vi "WILT Step Cooling Down.vi"(6 "Cool Down Period (seconds)":dbl=12.0 format="%#_13g", 7 "Station Number in":u32, 8 "Error In":errorcluster, 10 "Step 3 Input":T1, 11 "Dryer Step 5 In":T3 {"Night Cycle Count" format="%04d"; "Day Cycle Count" format="%04d"}) -> (0 "Error Out":errorcluster, 2 "Step 5 Output":T1, 3 "Dryer Step 5 Output":T3 {"Night Cycle Count" format="%04d"; "Day Cycle Count" format="%04d"})   [LabVIEW 2016]
uses:
  Type Definitions/WILT Station Test State Cluster.ctl
  Type Definitions/WILT Dryer Test State.ctl
  Type Definitions/WILT Dryer.ctl
  Type Definitions/WILT Dryer Details.ctl
  Type Definitions/WILT Agilent Channel Definition.ctl
  Type Definitions/WILT DAQ Data.ctl
  Globals/WILT Globals Main Program.vi
panel:
  # "Day"
  # "Night"
  # "Day"
  # "Night"
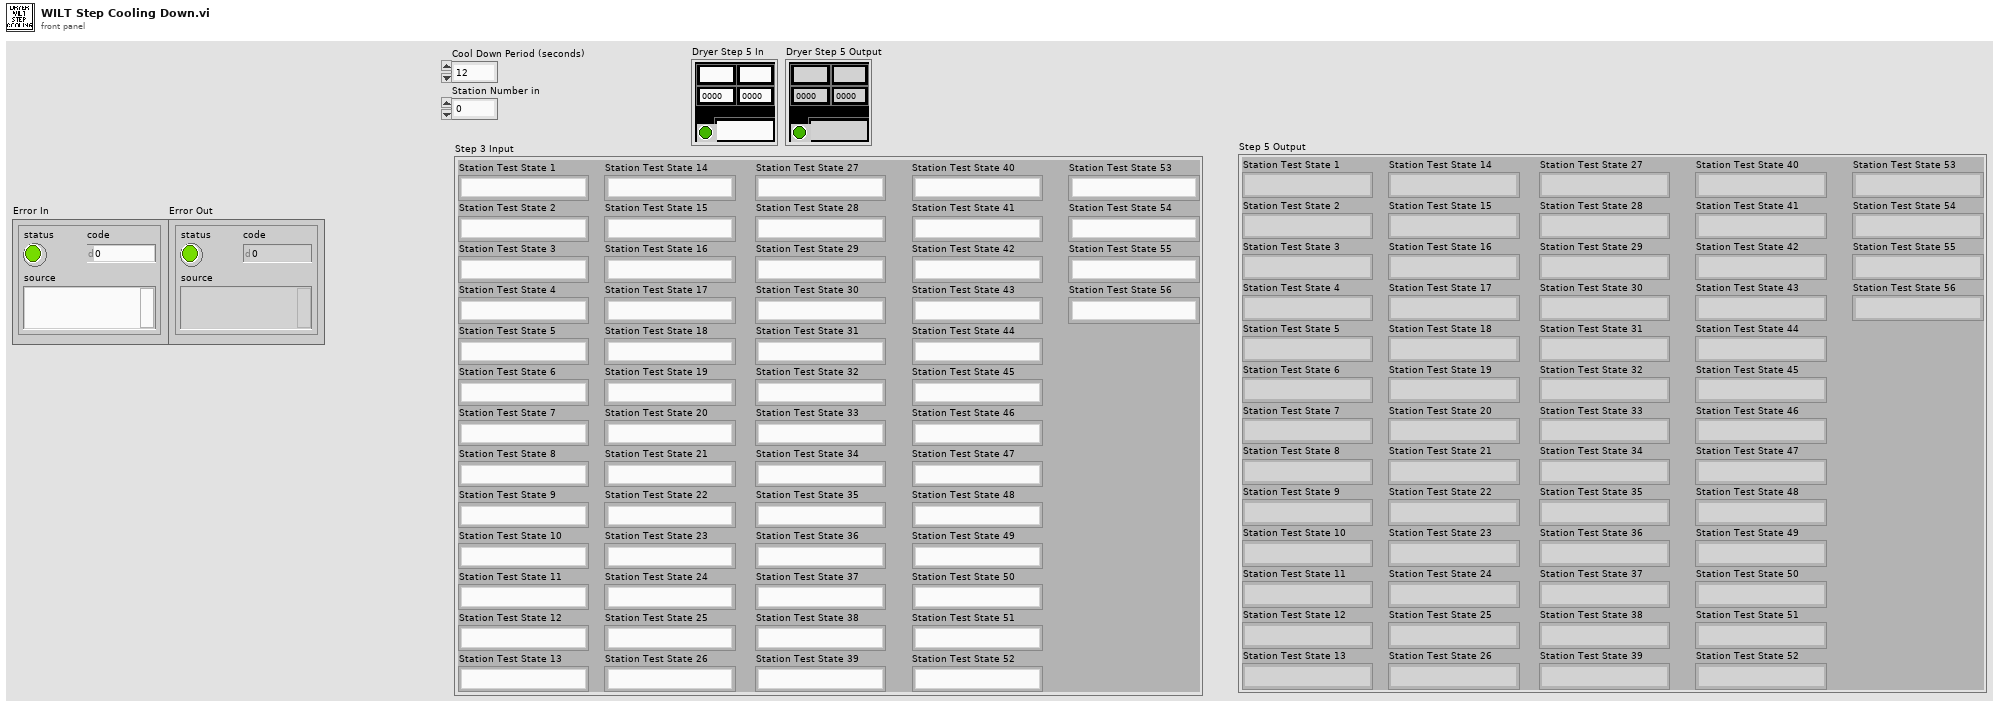
[diagram p1: front panel]
types:
  T1 = typedef "WILT Station Test State Cluster.ctl" = cluster{"Station Test State 1":T2, "Station Test State 2":T2, "Station Test State 3":T2, "Station Test State 4":T2, "Station Test State 5":T2, "Station Test State 6":T2, "Station Test State 7":T2, "Station Test State 8":T2, "Station Test State 9":T2, "Station Test State 10":T2, "Station Test State 11":T2, "Station Test State 12":T2, "Station Test State 13":T2, "Station Test State 14":T2, "Station Test State 15":T2, "Station Test State 16":T2, "Station Test State 17":T2, "Station Test State 18":T2, "Station Test State 19":T2, "Station Test State 20":T2, "Station Test State 21":T2, "Station Test State 22":T2, "Station Test State 23":T2, "Station Test State 24":T2, "Station Test State 25":T2, "Station Test State 26":T2, "Station Test State 27":T2, "Station Test State 28":T2, "Station Test State 29":T2, "Station Test State 30":T2, "Station Test State 31":T2, "Station Test State 32":T2, "Station Test State 33":T2, "Station Test State 34":T2, "Station Test State 35":T2, "Station Test State 36":T2, "Station Test State 37":T2, "Station Test State 38":T2, "Station Test State 39":T2, "Station Test State 40":T2, "Station Test State 41":T2, "Station Test State 42":T2, "Station Test State 43":T2, "Station Test State 44":T2, "Station Test State 45":T2, "Station Test State 46":T2, "Station Test State 47":T2, "Station Test State 48":T2, "Station Test State 49":T2, "Station Test State 50":T2, "Station Test State 51":T2, "Station Test State 52":T2, "Station Test State 53":T2, "Station Test State 54":T2, "Station Test State 55":T2, "Station Test State 56":T2}
  T2 = typedef "WILT Dryer Test State.ctl" = enum16{"No Serial Number", "Waiting for Dryer To Start", "Drying Clothes", "Water Injection 1 (On)", "Water Injection 1 Timer", "Water Injection 1 (Off)", "Pause Dryer", "Sending Start Stop CMD", "Pause Dryer 2", "Sending Start Stop CMD 2", "Drying Clothes 2", "Water Injection 2 (On)", "Water Injection 2 Timer", "Water Injection 2 (Off)", "Drying Clothes 3", "Cooling Down", "Sending Start Stop CMD 3", "Increment Cycle"}
  T3 = typedef "WILT Dryer.ctl" = cluster{"Lab ID":string, "Day Cycle Count":i32, "Station Label":string, "Dryer Details":T4, "Status Color":u32, "Invisible Button":bool, "Night Cycle Count":i32, "Station Index":i32, "Cycle Index":string, "Audit Alert":bool, "Agilent Channel Definition":T5, "DAQ Data":T6}
  T4 = typedef "WILT Dryer Details.ctl" = cluster{"Station":string, "Lab ID":string, "TR Number":string}
  T5 = typedef "WILT Agilent Channel Definition.ctl" = cluster{"Channel":string, "Station":string, "Label":string, "Agilent Station":string, "Data":dbl}
  T6 = typedef "WILT DAQ Data.ctl" = cluster{"L1 Current":dbl, "L2 Current":dbl, "Temperature  Deg F (TC)":dbl, "Volts":dbl, "Volts (208)":dbl, "SW (208)":dbl}
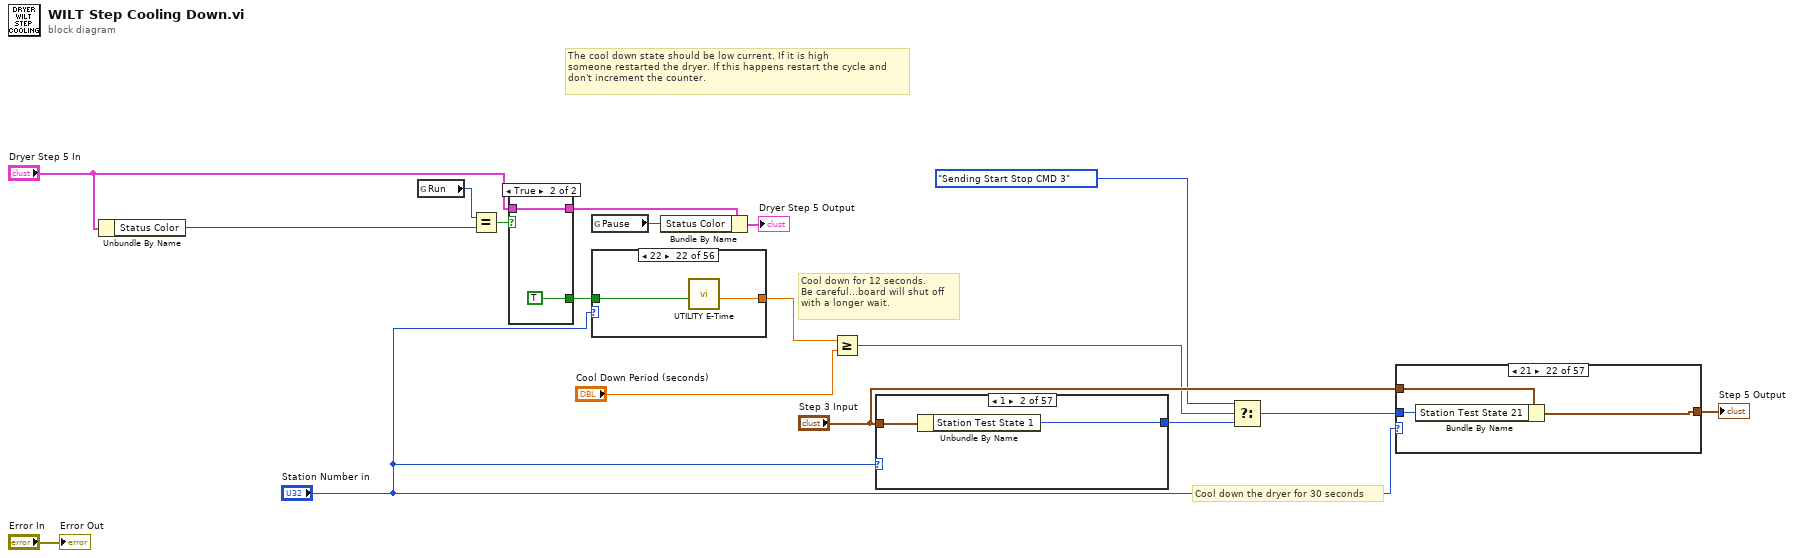
[diagram p0: block diagram]
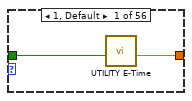
[diagram p2: hidden frame]
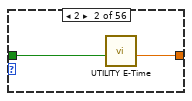
[diagram p3: hidden frame]
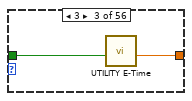
[diagram p4: hidden frame]
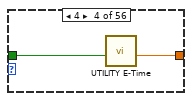
[diagram p5: hidden frame]
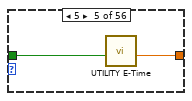
[diagram p6: hidden frame]
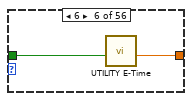
[diagram p7: hidden frame]
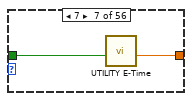
[diagram p8: hidden frame]
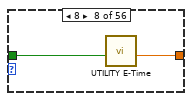
[diagram p9: hidden frame]
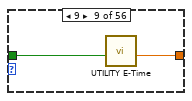
[diagram p10: hidden frame]
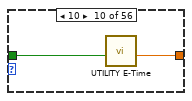
[diagram p11: hidden frame]
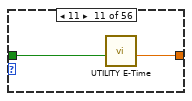
[diagram p12: hidden frame]
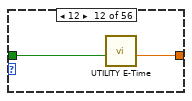
[diagram p13: hidden frame]
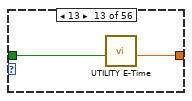
[diagram p14: hidden frame]
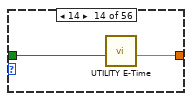
[diagram p15: hidden frame]
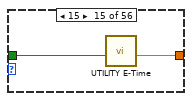
[diagram p16: hidden frame]
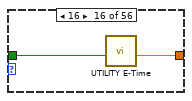
[diagram p17: hidden frame]
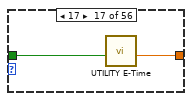
[diagram p18: hidden frame]
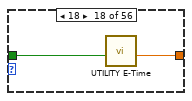
[diagram p19: hidden frame]
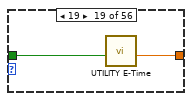
[diagram p20: hidden frame]
diagram:
  # "Cool down for 12 seconds.\nBe careful...board will shut off\nwith a longer wait."
  # "The cool down state should be low current. If it is high\nsomeone restarted the dryer. If this happens restart the cycle and\ndon't increment the counter."
  # "Cool down the dryer for 30 seconds"
  n1 = Unbundle By Name("Dryer Step 5 In") -> ("Status Color"=w13:u32)
  n2 = global read "WILT Globals Main Program.vi" "Run"() -> (w5:u32)
  n3 = Equal?(x=w5, y=w13) -> (x = y?=w4:bool)
  n4 = case shown="True" w4 {
    tunnel: [FALSE TRUE] -> w3
    tunnel: "Dryer Step 5 In" -> [w19 w21]
    tunnel: [w19 w21] -> w2
    frame False {
    }
    frame True {
    }
  }
  n5 = global read "WILT Globals Main Program.vi" "Pause"() -> (w1:u32)
  n6 = case shown="22" "Station Number in" {
    tunnel: [w24 w25 w27 w29 w31 w33 w35 w37 w39 w41 w43 w45 w47 w49 w51 w53 w55 w57 w59 w61 w63 w65 w67 w69 w71 w73 w75 w77 w79 w81 w83 w85 w87 w89 w91 w93 w95 w97 w99 w101 w103 w105 w107 w109 w111 w113 w115 w117 w119 w121 w123 w125 w127 w129 w131 w133] -> w7
    tunnel: w3 -> [w23 w26 w28 w30 w32 w34 w36 w38 w40 w42 w44 w46 w48 w50 w52 w54 w56 w58 w60 w62 w64 w66 w68 w70 w72 w74 w76 w78 w80 w82 w84 w86 w88 w90 w92 w94 w96 w98 w100 w102 w104 w106 w108 w110 w112 w114 w116 w118 w120 w122 w124 w126 w128 w130 w132 w134]
    frame 1, Default {
      n7 = call "UTILITY E-Time.vi"("Reset"=w23) -> ("Elapsed Time (sec)"=w24:dbl)  [unwired: 8 in, 2 out]
    }
    frame 2 {
      n8 = call "UTILITY E-Time.vi"("Reset"=w26) -> ("Elapsed Time (sec)"=w25:dbl)  [unwired: 8 in, 2 out]
    }
    frame 3 {
      n9 = call "UTILITY E-Time.vi"("Reset"=w28) -> ("Elapsed Time (sec)"=w27:dbl)  [unwired: 8 in, 2 out]
    }
    frame 4 {
      n10 = call "UTILITY E-Time.vi"("Reset"=w30) -> ("Elapsed Time (sec)"=w29:dbl)  [unwired: 8 in, 2 out]
    }
    frame 5 {
      n11 = call "UTILITY E-Time.vi"("Reset"=w32) -> ("Elapsed Time (sec)"=w31:dbl)  [unwired: 8 in, 2 out]
    }
    frame 6 {
      n12 = call "UTILITY E-Time.vi"("Reset"=w34) -> ("Elapsed Time (sec)"=w33:dbl)  [unwired: 8 in, 2 out]
    }
    frame 7 {
      n13 = call "UTILITY E-Time.vi"("Reset"=w36) -> ("Elapsed Time (sec)"=w35:dbl)  [unwired: 8 in, 2 out]
    }
    frame 8 {
      n14 = call "UTILITY E-Time.vi"("Reset"=w38) -> ("Elapsed Time (sec)"=w37:dbl)  [unwired: 8 in, 2 out]
    }
    frame 9 {
      n15 = call "UTILITY E-Time.vi"("Reset"=w40) -> ("Elapsed Time (sec)"=w39:dbl)  [unwired: 8 in, 2 out]
    }
    frame 10 {
      n16 = call "UTILITY E-Time.vi"("Reset"=w42) -> ("Elapsed Time (sec)"=w41:dbl)  [unwired: 8 in, 2 out]
    }
    frame 11 {
      n17 = call "UTILITY E-Time.vi"("Reset"=w44) -> ("Elapsed Time (sec)"=w43:dbl)  [unwired: 8 in, 2 out]
    }
    frame 12 {
      n18 = call "UTILITY E-Time.vi"("Reset"=w46) -> ("Elapsed Time (sec)"=w45:dbl)  [unwired: 8 in, 2 out]
    }
    frame 13 {
      n19 = call "UTILITY E-Time.vi"("Reset"=w48) -> ("Elapsed Time (sec)"=w47:dbl)  [unwired: 8 in, 2 out]
    }
    frame 14 {
      n20 = call "UTILITY E-Time.vi"("Reset"=w50) -> ("Elapsed Time (sec)"=w49:dbl)  [unwired: 8 in, 2 out]
    }
    frame 15 {
      n21 = call "UTILITY E-Time.vi"("Reset"=w52) -> ("Elapsed Time (sec)"=w51:dbl)  [unwired: 8 in, 2 out]
    }
    frame 16 {
      n22 = call "UTILITY E-Time.vi"("Reset"=w54) -> ("Elapsed Time (sec)"=w53:dbl)  [unwired: 8 in, 2 out]
    }
    frame 17 {
      n23 = call "UTILITY E-Time.vi"("Reset"=w56) -> ("Elapsed Time (sec)"=w55:dbl)  [unwired: 8 in, 2 out]
    }
    frame 18 {
      n24 = call "UTILITY E-Time.vi"("Reset"=w58) -> ("Elapsed Time (sec)"=w57:dbl)  [unwired: 8 in, 2 out]
    }
    frame 19 {
      n25 = call "UTILITY E-Time.vi"("Reset"=w60) -> ("Elapsed Time (sec)"=w59:dbl)  [unwired: 8 in, 2 out]
    }
    frame 20 {
      n26 = call "UTILITY E-Time.vi"("Reset"=w62) -> ("Elapsed Time (sec)"=w61:dbl)  [unwired: 8 in, 2 out]
    }
    frame 21 {
      n27 = call "UTILITY E-Time.vi"("Reset"=w64) -> ("Elapsed Time (sec)"=w63:dbl)  [unwired: 8 in, 2 out]
    }
    frame 22 {
      n28 = call "UTILITY E-Time.vi"("Reset"=w66) -> ("Elapsed Time (sec)"=w65:dbl)  [unwired: 8 in, 2 out]
    }
    frame 23 {
      n29 = call "UTILITY E-Time.vi"("Reset"=w68) -> ("Elapsed Time (sec)"=w67:dbl)  [unwired: 8 in, 2 out]
    }
    frame 24 {
      n30 = call "UTILITY E-Time.vi"("Reset"=w70) -> ("Elapsed Time (sec)"=w69:dbl)  [unwired: 8 in, 2 out]
    }
    frame 25 {
      n31 = call "UTILITY E-Time.vi"("Reset"=w72) -> ("Elapsed Time (sec)"=w71:dbl)  [unwired: 8 in, 2 out]
    }
    frame 26 {
      n32 = call "UTILITY E-Time.vi"("Reset"=w74) -> ("Elapsed Time (sec)"=w73:dbl)  [unwired: 8 in, 2 out]
    }
    frame 27 {
      n33 = call "UTILITY E-Time.vi"("Reset"=w76) -> ("Elapsed Time (sec)"=w75:dbl)  [unwired: 8 in, 2 out]
    }
    frame 28 {
      n34 = call "UTILITY E-Time.vi"("Reset"=w78) -> ("Elapsed Time (sec)"=w77:dbl)  [unwired: 8 in, 2 out]
    }
    frame 29 {
      n35 = call "UTILITY E-Time.vi"("Reset"=w80) -> ("Elapsed Time (sec)"=w79:dbl)  [unwired: 8 in, 2 out]
    }
    frame 30 {
      n36 = call "UTILITY E-Time.vi"("Reset"=w82) -> ("Elapsed Time (sec)"=w81:dbl)  [unwired: 8 in, 2 out]
    }
    frame 31 {
      n37 = call "UTILITY E-Time.vi"("Reset"=w84) -> ("Elapsed Time (sec)"=w83:dbl)  [unwired: 8 in, 2 out]
    }
    frame 32 {
      n38 = call "UTILITY E-Time.vi"("Reset"=w86) -> ("Elapsed Time (sec)"=w85:dbl)  [unwired: 8 in, 2 out]
    }
    frame 33 {
      n39 = call "UTILITY E-Time.vi"("Reset"=w88) -> ("Elapsed Time (sec)"=w87:dbl)  [unwired: 8 in, 2 out]
    }
    frame 34 {
      n40 = call "UTILITY E-Time.vi"("Reset"=w90) -> ("Elapsed Time (sec)"=w89:dbl)  [unwired: 8 in, 2 out]
    }
    frame 35 {
      n41 = call "UTILITY E-Time.vi"("Reset"=w92) -> ("Elapsed Time (sec)"=w91:dbl)  [unwired: 8 in, 2 out]
    }
    frame 36 {
      n42 = call "UTILITY E-Time.vi"("Reset"=w94) -> ("Elapsed Time (sec)"=w93:dbl)  [unwired: 8 in, 2 out]
    }
    frame 37 {
      n43 = call "UTILITY E-Time.vi"("Reset"=w96) -> ("Elapsed Time (sec)"=w95:dbl)  [unwired: 8 in, 2 out]
    }
    frame 38 {
      n44 = call "UTILITY E-Time.vi"("Reset"=w98) -> ("Elapsed Time (sec)"=w97:dbl)  [unwired: 8 in, 2 out]
    }
    frame 39 {
      n45 = call "UTILITY E-Time.vi"("Reset"=w100) -> ("Elapsed Time (sec)"=w99:dbl)  [unwired: 8 in, 2 out]
    }
    frame 40 {
      n46 = call "UTILITY E-Time.vi"("Reset"=w102) -> ("Elapsed Time (sec)"=w101:dbl)  [unwired: 8 in, 2 out]
    }
    frame 41 {
      n47 = call "UTILITY E-Time.vi"("Reset"=w104) -> ("Elapsed Time (sec)"=w103:dbl)  [unwired: 8 in, 2 out]
    }
    frame 42 {
      n48 = call "UTILITY E-Time.vi"("Reset"=w106) -> ("Elapsed Time (sec)"=w105:dbl)  [unwired: 8 in, 2 out]
    }
    frame 43 {
      n49 = call "UTILITY E-Time.vi"("Reset"=w108) -> ("Elapsed Time (sec)"=w107:dbl)  [unwired: 8 in, 2 out]
    }
    frame 44 {
      n50 = call "UTILITY E-Time.vi"("Reset"=w110) -> ("Elapsed Time (sec)"=w109:dbl)  [unwired: 8 in, 2 out]
    }
    frame 45 {
      n51 = call "UTILITY E-Time.vi"("Reset"=w112) -> ("Elapsed Time (sec)"=w111:dbl)  [unwired: 8 in, 2 out]
    }
    frame 46 {
      n52 = call "UTILITY E-Time.vi"("Reset"=w114) -> ("Elapsed Time (sec)"=w113:dbl)  [unwired: 8 in, 2 out]
    }
    frame 47 {
      n53 = call "UTILITY E-Time.vi"("Reset"=w116) -> ("Elapsed Time (sec)"=w115:dbl)  [unwired: 8 in, 2 out]
    }
    frame 48 {
      n54 = call "UTILITY E-Time.vi"("Reset"=w118) -> ("Elapsed Time (sec)"=w117:dbl)  [unwired: 8 in, 2 out]
    }
    frame 49 {
      n55 = call "UTILITY E-Time.vi"("Reset"=w120) -> ("Elapsed Time (sec)"=w119:dbl)  [unwired: 8 in, 2 out]
    }
    frame 50 {
      n56 = call "UTILITY E-Time.vi"("Reset"=w122) -> ("Elapsed Time (sec)"=w121:dbl)  [unwired: 8 in, 2 out]
    }
    frame 51 {
      n57 = call "UTILITY E-Time.vi"("Reset"=w124) -> ("Elapsed Time (sec)"=w123:dbl)  [unwired: 8 in, 2 out]
    }
    frame 52 {
      n58 = call "UTILITY E-Time.vi"("Reset"=w126) -> ("Elapsed Time (sec)"=w125:dbl)  [unwired: 8 in, 2 out]
    }
    frame 53 {
      n59 = call "UTILITY E-Time.vi"("Reset"=w128) -> ("Elapsed Time (sec)"=w127:dbl)  [unwired: 8 in, 2 out]
    }
    frame 54 {
      n60 = call "UTILITY E-Time.vi"("Reset"=w130) -> ("Elapsed Time (sec)"=w129:dbl)  [unwired: 8 in, 2 out]
    }
    frame 55 {
      n61 = call "UTILITY E-Time.vi"("Reset"=w132) -> ("Elapsed Time (sec)"=w131:dbl)  [unwired: 8 in, 2 out]
    }
    frame 56 {
      n62 = call "UTILITY E-Time.vi"("Reset"=w134) -> ("Elapsed Time (sec)"=w133:dbl)  [unwired: 8 in, 2 out]
    }
  }
  n63 = Bundle By Name(cluster=w2, "Status Color"=w1) -> (→"Dryer Step 5 Output":T3)
  n64 = Greater Or Equal?(x=w7, y="Cool Down Period (seconds)") -> (x >= y?=w14:bool)
  n65 = case shown="1" "Station Number in" {
    tunnel: "Step 3 Input" -> [_ w137 w139 w141 w143 w145 w147 w149 w151 w153 w155 w157 w159 w161 w163 w165 w167 w169 w171 w173 w175 w177 w179 w181 w183 w185 w187 w189 w191 w193 w195 w197 w199 w201 w203 w205 w207 w209 w211 w213 w215 w217 w219 w221 w223 w225 w227 w229 w231 w233 w235 w237 w239 w241 w243 w245 w247]
    tunnel: [WILT_Dryer_Test_State."No Serial Number" ("Station Test State 56") w136 w138 w140 w142 w144 w146 w148 w150 w152 w154 w156 w158 w160 w162 w164 w166 w168 w170 w172 w174 w176 w178 w180 w182 w184 w186 w188 w190 w192 w194 w196 w198 w200 w202 w204 w206 w208 w210 w212 w214 w216 w218 w220 w222 w224 w226 w228 w230 w232 w234 w236 w238 w240 w242 w244 w246] -> w18
    frame 0, Default {
      # "This is not a station.\nDo nothing"
    }
    frame 1 {
      n66 = Unbundle By Name(w137) -> ("Station Test State 1"=w136:T2)
    }
    frame 2 {
      n67 = Unbundle By Name(w139) -> ("Station Test State 2"=w138:T2)
    }
    frame 3 {
      n68 = Unbundle By Name(w141) -> ("Station Test State 3"=w140:T2)
    }
    frame 4 {
      n69 = Unbundle By Name(w143) -> ("Station Test State 4"=w142:T2)
    }
    frame 5 {
      n70 = Unbundle By Name(w145) -> ("Station Test State 5"=w144:T2)
    }
    frame 6 {
      n71 = Unbundle By Name(w147) -> ("Station Test State 6"=w146:T2)
    }
    frame 7 {
      n72 = Unbundle By Name(w149) -> ("Station Test State 7"=w148:T2)
    }
    frame 8 {
      n73 = Unbundle By Name(w151) -> ("Station Test State 8"=w150:T2)
    }
    frame 9 {
      n74 = Unbundle By Name(w153) -> ("Station Test State 9"=w152:T2)
    }
    frame 10 {
      n75 = Unbundle By Name(w155) -> ("Station Test State 10"=w154:T2)
    }
    frame 11 {
      n76 = Unbundle By Name(w157) -> ("Station Test State 11"=w156:T2)
    }
    frame 12 {
      n77 = Unbundle By Name(w159) -> ("Station Test State 12"=w158:T2)
    }
    frame 13 {
      n78 = Unbundle By Name(w161) -> ("Station Test State 13"=w160:T2)
    }
    frame 14 {
      n79 = Unbundle By Name(w163) -> ("Station Test State 14"=w162:T2)
    }
    frame 15 {
      n80 = Unbundle By Name(w165) -> ("Station Test State 15"=w164:T2)
    }
    frame 16 {
      n81 = Unbundle By Name(w167) -> ("Station Test State 16"=w166:T2)
    }
    frame 17 {
      n82 = Unbundle By Name(w169) -> ("Station Test State 17"=w168:T2)
    }
    frame 18 {
      n83 = Unbundle By Name(w171) -> ("Station Test State 18"=w170:T2)
    }
    frame 19 {
      n84 = Unbundle By Name(w173) -> ("Station Test State 19"=w172:T2)
    }
    frame 20 {
      n85 = Unbundle By Name(w175) -> ("Station Test State 20"=w174:T2)
    }
    frame 21 {
      n86 = Unbundle By Name(w177) -> ("Station Test State 21"=w176:T2)
    }
    frame 22 {
      n87 = Unbundle By Name(w179) -> ("Station Test State 22"=w178:T2)
    }
    frame 23 {
      n88 = Unbundle By Name(w181) -> ("Station Test State 23"=w180:T2)
    }
    frame 24 {
      n89 = Unbundle By Name(w183) -> ("Station Test State 24"=w182:T2)
    }
    frame 25 {
      n90 = Unbundle By Name(w185) -> ("Station Test State 25"=w184:T2)
    }
    frame 26 {
      n91 = Unbundle By Name(w187) -> ("Station Test State 26"=w186:T2)
    }
    frame 27 {
      n92 = Unbundle By Name(w189) -> ("Station Test State 27"=w188:T2)
    }
    frame 28 {
      n93 = Unbundle By Name(w191) -> ("Station Test State 28"=w190:T2)
    }
    frame 29 {
      n94 = Unbundle By Name(w193) -> ("Station Test State 29"=w192:T2)
    }
    frame 30 {
      n95 = Unbundle By Name(w195) -> ("Station Test State 30"=w194:T2)
    }
    frame 31 {
      n96 = Unbundle By Name(w197) -> ("Station Test State 31"=w196:T2)
    }
    frame 32 {
      n97 = Unbundle By Name(w199) -> ("Station Test State 32"=w198:T2)
    }
    frame 33 {
      n98 = Unbundle By Name(w201) -> ("Station Test State 33"=w200:T2)
    }
    frame 34 {
      n99 = Unbundle By Name(w203) -> ("Station Test State 34"=w202:T2)
    }
    frame 35 {
      n100 = Unbundle By Name(w205) -> ("Station Test State 35"=w204:T2)
    }
    frame 36 {
      n101 = Unbundle By Name(w207) -> ("Station Test State 36"=w206:T2)
    }
    frame 37 {
      n102 = Unbundle By Name(w209) -> ("Station Test State 37"=w208:T2)
    }
    frame 38 {
      n103 = Unbundle By Name(w211) -> ("Station Test State 38"=w210:T2)
    }
    frame 39 {
      n104 = Unbundle By Name(w213) -> ("Station Test State 39"=w212:T2)
    }
    frame 40 {
      n105 = Unbundle By Name(w215) -> ("Station Test State 40"=w214:T2)
    }
    frame 41 {
      n106 = Unbundle By Name(w217) -> ("Station Test State 41"=w216:T2)
    }
    frame 42 {
      n107 = Unbundle By Name(w219) -> ("Station Test State 42"=w218:T2)
    }
    frame 43 {
      n108 = Unbundle By Name(w221) -> ("Station Test State 43"=w220:T2)
    }
    frame 44 {
      n109 = Unbundle By Name(w223) -> ("Station Test State 44"=w222:T2)
    }
    frame 45 {
      n110 = Unbundle By Name(w225) -> ("Station Test State 45"=w224:T2)
    }
    frame 46 {
      n111 = Unbundle By Name(w227) -> ("Station Test State 46"=w226:T2)
    }
    frame 47 {
      n112 = Unbundle By Name(w229) -> ("Station Test State 47"=w228:T2)
    }
    frame 48 {
      n113 = Unbundle By Name(w231) -> ("Station Test State 48"=w230:T2)
    }
    frame 49 {
      n114 = Unbundle By Name(w233) -> ("Station Test State 49"=w232:T2)
    }
    frame 50 {
      n115 = Unbundle By Name(w235) -> ("Station Test State 50"=w234:T2)
    }
    frame 51 {
      n116 = Unbundle By Name(w237) -> ("Station Test State 51"=w236:T2)
    }
    frame 52 {
      n117 = Unbundle By Name(w239) -> ("Station Test State 52"=w238:T2)
    }
    frame 53 {
      n118 = Unbundle By Name(w241) -> ("Station Test State 53"=w240:T2)
    }
    frame 54 {
      n119 = Unbundle By Name(w243) -> ("Station Test State 54"=w242:T2)
    }
    frame 55 {
      n120 = Unbundle By Name(w245) -> ("Station Test State 55"=w244:T2)
    }
    frame 56 {
      n121 = Unbundle By Name(w247) -> ("Station Test State 56"=w246:T2)
    }
  }
  n122 = Select(t=WILT_Dryer_Test_State."Sending Start Stop CMD 3" ("Current State 2"), s=w14, f=w18) -> (s? t:f=w10:T2)
  n123 = case shown="21" "Station Number in" {
    tunnel: "Step 3 Input" -> [w248 w251 w254 w257 w260 w263 w266 w269 w272 w275 w278 w281 w284 w287 w290 w293 w296 w299 w302 w305 w308 w311 w314 w317 w320 w323 w326 w329 w332 w335 w338 w341 w344 w347 w350 w353 w356 w359 w362 w365 w368 w371 w374 w377 w380 w383 w386 w389 w392 w395 w398 w401 w404 w407 w410 w413 w416]
    tunnel: w10 -> [_ w250 w252 w255 w258 w261 w264 w267 w270 w273 w276 w279 w282 w285 w288 w291 w294 w297 w300 w303 w306 w309 w312 w315 w318 w321 w324 w327 w330 w333 w336 w339 w342 w345 w348 w351 w354 w357 w360 w363 w366 w369 w372 w375 w378 w381 w384 w387 w390 w393 w396 w399 w402 w405 w408 w411 w414]
    tunnel: [w248 w249 w253 w256 w259 w262 w265 w268 w271 w274 w277 w280 w283 w286 w289 w292 w295 w298 w301 w304 w307 w310 w313 w316 w319 w322 w325 w328 w331 w334 w337 w340 w343 w346 w349 w352 w355 w358 w361 w364 w367 w370 w373 w376 w379 w382 w385 w388 w391 w394 w397 w400 w403 w406 w409 w412 w415] -> w16
    frame 0, Default {
      # "Not a valid station. Do nothing"
    }
    frame 1 {
      n124 = Bundle By Name(cluster=w251, "Station Test State 1"=w250) -> (w249:T1)
    }
    frame 2 {
      n125 = Bundle By Name(cluster=w254, "Station Test State 2"=w252) -> (w253:T1)
    }
    frame 3 {
      n126 = Bundle By Name(cluster=w257, "Station Test State 3"=w255) -> (w256:T1)
    }
    frame 4 {
      n127 = Bundle By Name(cluster=w260, "Station Test State 4"=w258) -> (w259:T1)
    }
    frame 5 {
      n128 = Bundle By Name(cluster=w263, "Station Test State 5"=w261) -> (w262:T1)
    }
    frame 6 {
      n129 = Bundle By Name(cluster=w266, "Station Test State 6"=w264) -> (w265:T1)
    }
    frame 7 {
      n130 = Bundle By Name(cluster=w269, "Station Test State 7"=w267) -> (w268:T1)
    }
    frame 8 {
      n131 = Bundle By Name(cluster=w272, "Station Test State 8"=w270) -> (w271:T1)
    }
    frame 9 {
      n132 = Bundle By Name(cluster=w275, "Station Test State 9"=w273) -> (w274:T1)
    }
    frame 10 {
      n133 = Bundle By Name(cluster=w278, "Station Test State 10"=w276) -> (w277:T1)
    }
    frame 11 {
      n134 = Bundle By Name(cluster=w281, "Station Test State 11"=w279) -> (w280:T1)
    }
    frame 12 {
      n135 = Bundle By Name(cluster=w284, "Station Test State 12"=w282) -> (w283:T1)
    }
    frame 13 {
      n136 = Bundle By Name(cluster=w287, "Station Test State 13"=w285) -> (w286:T1)
    }
    frame 14 {
      n137 = Bundle By Name(cluster=w290, "Station Test State 14"=w288) -> (w289:T1)
    }
    frame 15 {
      n138 = Bundle By Name(cluster=w293, "Station Test State 15"=w291) -> (w292:T1)
    }
    frame 16 {
      n139 = Bundle By Name(cluster=w296, "Station Test State 16"=w294) -> (w295:T1)
    }
    frame 17 {
      n140 = Bundle By Name(cluster=w299, "Station Test State 17"=w297) -> (w298:T1)
    }
    frame 18 {
      n141 = Bundle By Name(cluster=w302, "Station Test State 18"=w300) -> (w301:T1)
    }
    frame 19 {
      n142 = Bundle By Name(cluster=w305, "Station Test State 19"=w303) -> (w304:T1)
    }
    frame 20 {
      n143 = Bundle By Name(cluster=w308, "Station Test State 20"=w306) -> (w307:T1)
    }
    frame 21 {
      n144 = Bundle By Name(cluster=w311, "Station Test State 21"=w309) -> (w310:T1)
    }
    frame 22 {
      n145 = Bundle By Name(cluster=w314, "Station Test State 22"=w312) -> (w313:T1)
    }
    frame 23 {
      n146 = Bundle By Name(cluster=w317, "Station Test State 23"=w315) -> (w316:T1)
    }
    frame 24 {
      n147 = Bundle By Name(cluster=w320, "Station Test State 24"=w318) -> (w319:T1)
    }
    frame 25 {
      n148 = Bundle By Name(cluster=w323, "Station Test State 25"=w321) -> (w322:T1)
    }
    frame 26 {
      n149 = Bundle By Name(cluster=w326, "Station Test State 26"=w324) -> (w325:T1)
    }
    frame 27 {
      n150 = Bundle By Name(cluster=w329, "Station Test State 27"=w327) -> (w328:T1)
    }
    frame 28 {
      n151 = Bundle By Name(cluster=w332, "Station Test State 28"=w330) -> (w331:T1)
    }
    frame 29 {
      n152 = Bundle By Name(cluster=w335, "Station Test State 29"=w333) -> (w334:T1)
    }
    frame 30 {
      n153 = Bundle By Name(cluster=w338, "Station Test State 30"=w336) -> (w337:T1)
    }
    frame 31 {
      n154 = Bundle By Name(cluster=w341, "Station Test State 31"=w339) -> (w340:T1)
    }
    frame 32 {
      n155 = Bundle By Name(cluster=w344, "Station Test State 32"=w342) -> (w343:T1)
    }
    frame 33 {
      n156 = Bundle By Name(cluster=w347, "Station Test State 33"=w345) -> (w346:T1)
    }
    frame 34 {
      n157 = Bundle By Name(cluster=w350, "Station Test State 34"=w348) -> (w349:T1)
    }
    frame 35 {
      n158 = Bundle By Name(cluster=w353, "Station Test State 35"=w351) -> (w352:T1)
    }
    frame 36 {
      n159 = Bundle By Name(cluster=w356, "Station Test State 36"=w354) -> (w355:T1)
    }
    frame 37 {
      n160 = Bundle By Name(cluster=w359, "Station Test State 37"=w357) -> (w358:T1)
    }
    frame 38 {
      n161 = Bundle By Name(cluster=w362, "Station Test State 38"=w360) -> (w361:T1)
    }
    frame 39 {
      n162 = Bundle By Name(cluster=w365, "Station Test State 39"=w363) -> (w364:T1)
    }
    frame 40 {
      n163 = Bundle By Name(cluster=w368, "Station Test State 40"=w366) -> (w367:T1)
    }
    frame 41 {
      n164 = Bundle By Name(cluster=w371, "Station Test State 41"=w369) -> (w370:T1)
    }
    frame 42 {
      n165 = Bundle By Name(cluster=w374, "Station Test State 42"=w372) -> (w373:T1)
    }
    frame 43 {
      n166 = Bundle By Name(cluster=w377, "Station Test State 43"=w375) -> (w376:T1)
    }
    frame 44 {
      n167 = Bundle By Name(cluster=w380, "Station Test State 44"=w378) -> (w379:T1)
    }
    frame 45 {
      n168 = Bundle By Name(cluster=w383, "Station Test State 45"=w381) -> (w382:T1)
    }
    frame 46 {
      n169 = Bundle By Name(cluster=w386, "Station Test State 46"=w384) -> (w385:T1)
    }
    frame 47 {
      n170 = Bundle By Name(cluster=w389, "Station Test State 47"=w387) -> (w388:T1)
    }
    frame 48 {
      n171 = Bundle By Name(cluster=w392, "Station Test State 48"=w390) -> (w391:T1)
    }
    frame 49 {
      n172 = Bundle By Name(cluster=w395, "Station Test State 49"=w393) -> (w394:T1)
    }
    frame 50 {
      n173 = Bundle By Name(cluster=w398, "Station Test State 50"=w396) -> (w397:T1)
    }
    frame 51 {
      n174 = Bundle By Name(cluster=w401, "Station Test State 51"=w399) -> (w400:T1)
    }
    frame 52 {
      n175 = Bundle By Name(cluster=w404, "Station Test State 52"=w402) -> (w403:T1)
    }
    frame 53 {
      n176 = Bundle By Name(cluster=w407, "Station Test State 53"=w405) -> (w406:T1)
    }
    frame 54 {
      n177 = Bundle By Name(cluster=w410, "Station Test State 54"=w408) -> (w409:T1)
    }
    frame 55 {
      n178 = Bundle By Name(cluster=w413, "Station Test State 55"=w411) -> (w412:T1)
    }
    frame 56 {
      n179 = Bundle By Name(cluster=w416, "Station Test State 56"=w414) -> (w415:T1)
    }
  }
  "Step 5 Output" <- w16
  "Error Out" <- "Error In"
